vi ".....GAIT RECOGNITION only.vi"() -> ()   [LabVIEW 2018]
uses:
  <vilib>/University of Leeds/Kinesthesia Toolkit for Microsoft Kinect/_Polymorphic Configure/Event-Skeleton and Video.vi
  <vilib>/Utility/file.llb/Read Delimited Spreadsheet (DBL).vi
  <vilib>/University of Leeds/Kinesthesia Toolkit for Microsoft Kinect/_Polymorphic Read/Read-Skeleton and Video.vi
  <vilib>/University of Leeds/Kinesthesia Toolkit for Microsoft Kinect/_Polymorphic Close/Close-Skeleton and Video.vi
panel:
  out "3D Skeleton":refnum<vi>(3d-picture)
  out "2D Picture":picture
  out "recognized??":bool
  out "real time bone length":dbl[](array[numeric])
  out "19 means":dbl[][](array[numeric])
  in  "file path":path=path "D:/mean.csv"
  out "score":dbl
  # "Skeleton Recognition System"
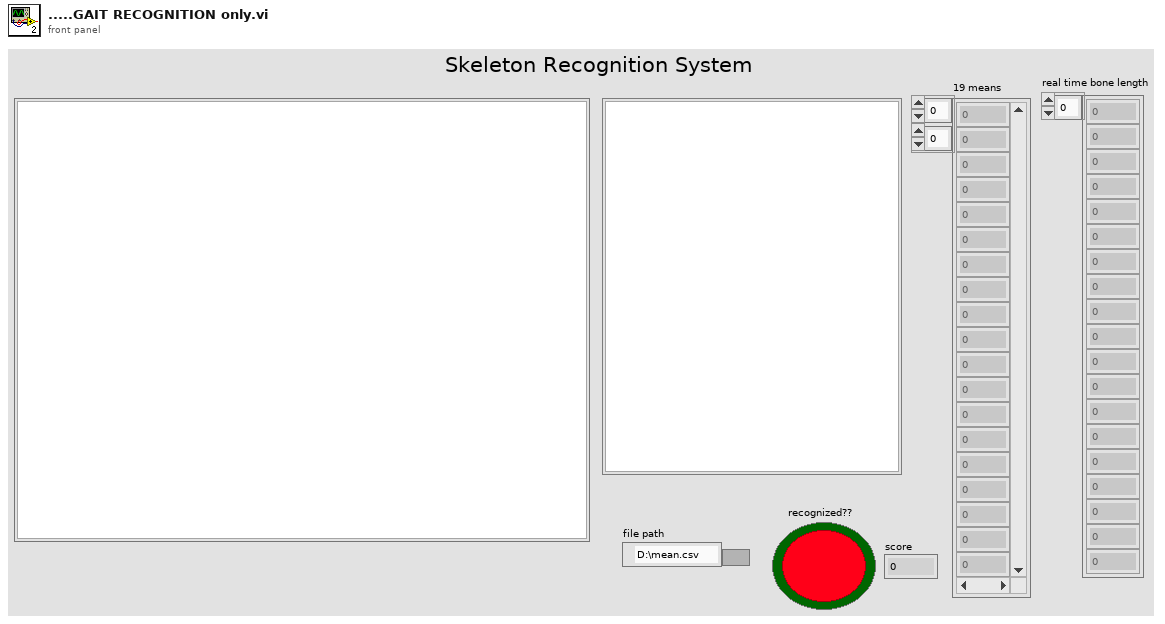
[diagram p1: front panel]
types:
  T1 = enum16{"hip centre", "spine", "shoulder centre", "head", "shoulder left", "elbow left", "wrist left", "hand left", "shoulder right", "elbow right", "wrist right", "hand right", "hip left", "knee left", "ankle left", "foot left", "hip right", "knee right", "ankle right", "foot right"}
  T2 = cluster{cluster{"reference out":refnum<k24>, "KinectSensors":refnum<k24>}, "get_Item":refnum<k24>}
  T3 = cluster{"reference out":refnum<k24>, "KinectSensors":refnum<k24>, "SkeletonStream":refnum<k24>, "ColorStream":refnum<k24>, refnum<k24>[], "get_Item":refnum<k24>}
  T4 = cluster{"Scene":refnum<vi>, "Joints":refnum<vi>[], "Bones":refnum<vi>[]}
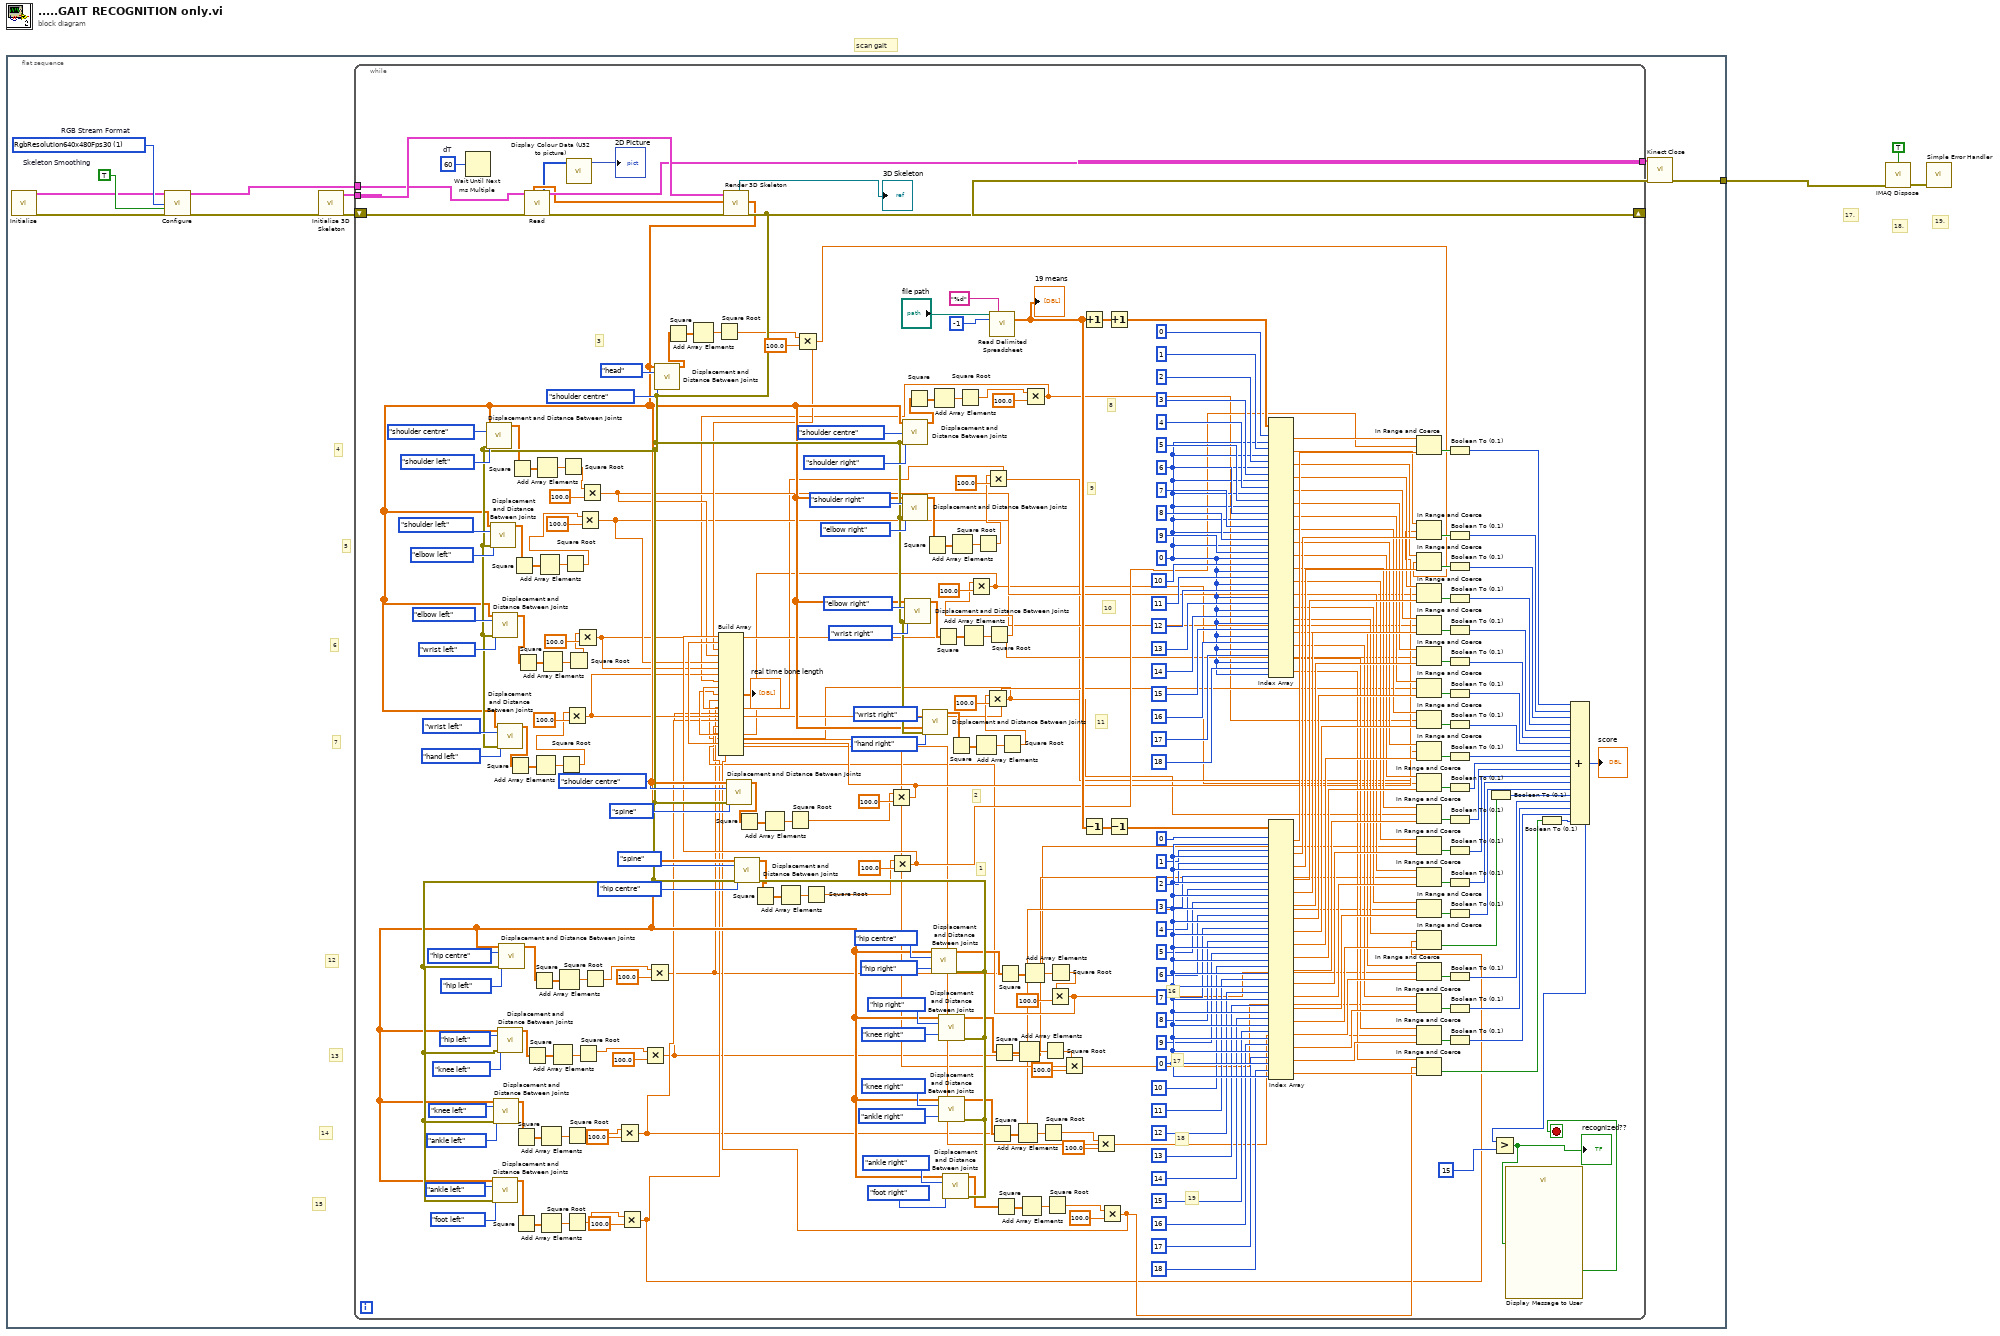
[diagram p0: block diagram]
diagram:
  # "19."
  # "17."
  # "18."
  # "scan gait"
  n1 = flat-sequence {
    tunnel: [w4] -> w1
    frame #0 {
      w10 = 1 items=["Undefined", "RgbResolution640x480Fps30", "RgbResolution1280x960Fps12", "YuvResolution640x480Fps15", "RawYuvResolution640x480Fps15"]  # RGB Stream Format
      w9 = TRUE  # Skeleton Smoothing
      # "15"
      # "14"
      # "13"
      # "12"
      # "7"
      # "6"
      # "5"
      # "4"
      n2 = call <vilib>:"Initialise.vi"() -> ("Kinect References out"=w5:T2, "error out"=w6:errorcluster)  [unwired: 14 in]
      n3 = call-poly <vilib>:"Configure.vi"("Kinect References in"=w5, "RGB Stream Format"=w10, "Skeleton Smoothing"=w9, "error in"=w6) -> ("Kinect References out"=w11:T3, "error out"=w12:errorcluster)  [unwired: 10 in]
      n4 = call <vilib>:"Initialise 3D Skeleton.vi"("error in (no error)"=w12) -> ("error out"=w13:errorcluster, "Scene & Skeleton Refs"=w14:T4)  [unwired: 9 in]
      n5 = while {
        tunnel: [w301] -> w7
        tunnel: w14 -> [w307]
        tunnel: w11 -> [w302]
        shift-right: [w260] -> w8
        shift-left: w13 -> [w304]
        stop <- w15 stop-if-true
        w136 = 0 ("disabled index (col)")
        w138 = 0 ("disabled index (col)")
        w305 = u32 60  # dT
        # "19"
        # "18"
        # "17"
        # "16"
        # "2"
        # "1"
        # "11"
        # "10"
        # "9"
        # "8"
        # "3"
        n6 = Wait Until Next ms Multiple(millisecond multiple=w305) -> ()  [unwired: 1 out]
        n7 = call-poly <vilib>:"Read.vi"("Kinect References in"=w302, "error in (no error)"=w304) -> ("Primary Skeleton Array"=w300:dbl[][], "Colour output array (U24, RGB)"=w299:u32[][], "Kinect References out"=w301:T3, "error out"=w303:errorcluster)  [unwired: 9 in, 1 out]
        n8 = call <vilib>:"Display Colour Data (U32 to picture).vi"("Colour output array (U24, RGB)"=w299) -> ("new picture"=→"2D Picture":picture)  [unwired: 10 in]
        n9 = call <vilib>:"Render 3D Skeleton.vi"("error in (no error)"=w303, "Array of Joint Positions"=w300, "Scene & Skeleton Refs In"=w307) -> ("error out"=w260:errorcluster, "Array of Joint Positions Out"=w259:dbl[][], "Scene Out"=→"3D Skeleton":refnum<vi>)  [unwired: 5 in, 1 out]
        n10 = call <vilib>:"Displacement and Distance Between Joints.vi"("Array of Joint Positions"=w259, "Joint 1"=T1."shoulder centre", "Joint 2"=T1."shoulder left", "error in (no error)"=w260) -> ("X Y Z Displacement Between Joints 1 and 2"=w250:dbl[])  [unwired: 10 in, 1 out]
        n11 = call <vilib>:"Displacement and Distance Between Joints.vi"("Array of Joint Positions"=w259, "Joint 1"=T1."shoulder left", "Joint 2"=T1."elbow left", "error in (no error)"=w260) -> ("X Y Z Displacement Between Joints 1 and 2"=w247:dbl[])  [unwired: 10 in, 1 out]
        n12 = call <vilib>:"Displacement and Distance Between Joints.vi"("Array of Joint Positions"=w259, "Joint 1"=T1."elbow left", "Joint 2"=T1."wrist left", "error in (no error)"=w260) -> ("X Y Z Displacement Between Joints 1 and 2"=w241:dbl[])  [unwired: 10 in, 1 out]
        n13 = call <vilib>:"Displacement and Distance Between Joints.vi"("Array of Joint Positions"=w259, "Joint 1"=T1."ankle left", "Joint 2"=T1."foot left", "error in (no error)"=w260) -> ("X Y Z Displacement Between Joints 1 and 2"=w214:dbl[])  [unwired: 10 in, 1 out]
        n14 = call <vilib>:"Displacement and Distance Between Joints.vi"("Array of Joint Positions"=w259, "Joint 1"=T1."knee left", "Joint 2"=T1."ankle left", "error in (no error)"=w260) -> ("X Y Z Displacement Between Joints 1 and 2"=w215:dbl[])  [unwired: 10 in, 1 out]
        n15 = call <vilib>:"Displacement and Distance Between Joints.vi"("Array of Joint Positions"=w259, "Joint 1"=T1."wrist left", "Joint 2"=T1."hand left", "error in (no error)"=w260) -> ("X Y Z Displacement Between Joints 1 and 2"=w231:dbl[])  [unwired: 10 in, 1 out]
        n16 = call <vilib>:"Displacement and Distance Between Joints.vi"("Array of Joint Positions"=w259, "Joint 1"=T1."hip left", "Joint 2"=T1."knee left", "error in (no error)"=w260) -> ("X Y Z Displacement Between Joints 1 and 2"=w216:dbl[])  [unwired: 10 in, 1 out]
        n17 = call <vilib>:"Displacement and Distance Between Joints.vi"("Array of Joint Positions"=w259, "Joint 1"=T1."hip centre", "Joint 2"=T1."hip left", "error in (no error)"=w260) -> ("X Y Z Displacement Between Joints 1 and 2"=w223:dbl[])  [unwired: 10 in, 1 out]
        n18 = Square(x=w231) -> (x^2=w235:dbl[])
        n19 = Square(x=w250) -> (x^2=w252:dbl[])
        n20 = Square(x=w247) -> (x^2=w249:dbl[])
        n21 = Square(x=w215) -> (x^2=w220:dbl[])
        n22 = Square(x=w214) -> (x^2=w218:dbl[])
        n23 = Square(x=w241) -> (x^2=w243:dbl[])
        n24 = Square(x=w216) -> (x^2=w222:dbl[])
        n25 = Square(x=w223) -> (x^2=w225:dbl[])
        n26 = Add Array Elements(numeric array=w235) -> (sum=w234:dbl)
        n27 = Add Array Elements(numeric array=w252) -> (sum=w251:dbl)
        n28 = Add Array Elements(numeric array=w249) -> (sum=w248:dbl)
        n29 = Add Array Elements(numeric array=w220) -> (sum=w219:dbl)
        n30 = Add Array Elements(numeric array=w218) -> (sum=w217:dbl)
        n31 = Add Array Elements(numeric array=w243) -> (sum=w242:dbl)
        n32 = Add Array Elements(numeric array=w222) -> (sum=w221:dbl)
        n33 = Add Array Elements(numeric array=w225) -> (sum=w224:dbl)
        n34 = Square Root(x=w234) -> (sqrt(x)=w190:dbl)
        n35 = Square Root(x=w251) -> (sqrt(x)=w198:dbl)
        n36 = Square Root(x=w248) -> (sqrt(x)=w194:dbl)
        n37 = Multiply(x=w190, y=100.0) -> (x*y=w29:dbl)
        n38 = Square Root(x=w219) -> (sqrt(x)=w172:dbl)
        n39 = Square Root(x=w217) -> (sqrt(x)=w170:dbl)
        n40 = Square Root(x=w242) -> (sqrt(x)=w192:dbl)
        n41 = Multiply(x=w192, y=100.0) -> (x*y=w30:dbl)
        n42 = Square Root(x=w221) -> (sqrt(x)=w174:dbl)
        n43 = Multiply(x=w194, y=100.0) -> (x*y=w31:dbl)
        n44 = Multiply(x=w198, y=100.0) -> (x*y=w32:dbl)
        n45 = Square Root(x=w224) -> (sqrt(x)=w176:dbl)
        n46 = Multiply(x=w172, y=100.0) -> (x*y=w20:dbl)
        n47 = Multiply(x=w170, y=100.0) -> (x*y=w21:dbl)
        n48 = Multiply(x=w174, y=100.0) -> (x*y=w19:dbl)
        n49 = Multiply(x=w176, y=100.0) -> (x*y=w18:dbl)
        n50 = call <vilib>:"Displacement and Distance Between Joints.vi"("Array of Joint Positions"=w259, "Joint 1"=T1."head", "Joint 2"=T1."shoulder centre", "error in (no error)"=w260) -> ("X Y Z Displacement Between Joints 1 and 2"=w256:dbl[])  [unwired: 10 in, 1 out]
        n51 = Square(x=w256) -> (x^2=w258:dbl[])
        n52 = Add Array Elements(numeric array=w258) -> (sum=w257:dbl)
        n53 = Square Root(x=w257) -> (sqrt(x)=w196:dbl)
        n54 = call <vilib>:"Displacement and Distance Between Joints.vi"("Array of Joint Positions"=w259, "Joint 1"=T1."shoulder centre", "Joint 2"=T1."spine", "error in (no error)"=w260) -> ("X Y Z Displacement Between Joints 1 and 2"=w229:dbl[])  [unwired: 10 in, 1 out]
        n55 = call <vilib>:"Displacement and Distance Between Joints.vi"("Array of Joint Positions"=w259, "Joint 1"=T1."spine", "Joint 2"=T1."hip centre", "error in (no error)"=w260) -> ("X Y Z Displacement Between Joints 1 and 2"=w226:dbl[])  [unwired: 10 in, 1 out]
        n56 = Square(x=w229) -> (x^2=w237:dbl[])
        n57 = Square(x=w226) -> (x^2=w228:dbl[])
        n58 = Add Array Elements(numeric array=w237) -> (sum=w236:dbl)
        n59 = Add Array Elements(numeric array=w228) -> (sum=w227:dbl)
        n60 = Square Root(x=w236) -> (sqrt(x)=w188:dbl)
        n61 = Multiply(x=w196, y=100.0) -> (x*y=w33:dbl)
        n62 = Square Root(x=w227) -> (sqrt(x)=w178:dbl)
        n63 = Multiply(x=w188, y=100.0) -> (x*y=w34:dbl)
        n64 = Multiply(x=w178, y=100.0) -> (x*y=w35:dbl)
        n65 = call <vilib>:"Displacement and Distance Between Joints.vi"("Array of Joint Positions"=w259, "Joint 1"=T1."shoulder centre", "Joint 2"=T1."shoulder right", "error in (no error)"=w260) -> ("X Y Z Displacement Between Joints 1 and 2"=w253:dbl[])  [unwired: 10 in, 1 out]
        n66 = call <vilib>:"Displacement and Distance Between Joints.vi"("Array of Joint Positions"=w259, "Joint 1"=T1."shoulder right", "Joint 2"=T1."elbow right", "error in (no error)"=w260) -> ("X Y Z Displacement Between Joints 1 and 2"=w244:dbl[])  [unwired: 10 in, 1 out]
        n67 = call <vilib>:"Displacement and Distance Between Joints.vi"("Array of Joint Positions"=w259, "Joint 1"=T1."elbow right", "Joint 2"=T1."wrist right", "error in (no error)"=w260) -> ("X Y Z Displacement Between Joints 1 and 2"=w238:dbl[])  [unwired: 10 in, 1 out]
        n68 = Square(x=w253) -> (x^2=w255:dbl[])
        n69 = call <vilib>:"Displacement and Distance Between Joints.vi"("Array of Joint Positions"=w259, "Joint 1"=T1."wrist right", "Joint 2"=T1."hand right", "error in (no error)"=w260) -> ("X Y Z Displacement Between Joints 1 and 2"=w230:dbl[])  [unwired: 10 in, 1 out]
        n70 = Square(x=w244) -> (x^2=w246:dbl[])
        n71 = Add Array Elements(numeric array=w255) -> (sum=w254:dbl)
        n72 = call <vilib>:"Displacement and Distance Between Joints.vi"("Array of Joint Positions"=w259, "Joint 1"=T1."hip centre", "Joint 2"=T1."hip right", "error in (no error)"=w260) -> ("X Y Z Displacement Between Joints 1 and 2"=w211:dbl[])  [unwired: 10 in, 1 out]
        n73 = Square(x=w238) -> (x^2=w240:dbl[])
        n74 = call <vilib>:"Displacement and Distance Between Joints.vi"("Array of Joint Positions"=w259, "Joint 1"=T1."hip right", "Joint 2"=T1."knee right", "error in (no error)"=w260) -> ("X Y Z Displacement Between Joints 1 and 2"=w204:dbl[])  [unwired: 10 in, 1 out]
        n75 = call <vilib>:"Displacement and Distance Between Joints.vi"("Array of Joint Positions"=w259, "Joint 1"=T1."knee right", "Joint 2"=T1."ankle right", "error in (no error)"=w260) -> ("X Y Z Displacement Between Joints 1 and 2"=w203:dbl[])  [unwired: 10 in, 1 out]
        n76 = call <vilib>:"Displacement and Distance Between Joints.vi"("Array of Joint Positions"=w259, "Joint 1"=T1."ankle right", "Joint 2"=T1."foot right", "error in (no error)"=w260) -> ("X Y Z Displacement Between Joints 1 and 2"=w202:dbl[])  [unwired: 10 in, 1 out]
        n77 = Square(x=w230) -> (x^2=w233:dbl[])
        n78 = Add Array Elements(numeric array=w246) -> (sum=w245:dbl)
        n79 = Square Root(x=w254) -> (sqrt(x)=w186:dbl)
        n80 = Add Array Elements(numeric array=w240) -> (sum=w239:dbl)
        n81 = Add Array Elements(numeric array=w233) -> (sum=w232:dbl)
        n82 = Square Root(x=w245) -> (sqrt(x)=w184:dbl)
        n83 = Multiply(x=w184, y=100.0) -> (x*y=w27:dbl)
        n84 = Square Root(x=w239) -> (sqrt(x)=w182:dbl)
        n85 = Multiply(x=w182, y=100.0) -> (x*y=w26:dbl)
        n86 = call-poly <vilib>:"Read Delimited Spreadsheet.vi"("file path (dialog if empty)"="file path", "format (%.3f)"="%d", "number of rows (all:-1)"=-1) -> ("all rows"=w114:dbl[][])  [unwired: 7 in, 5 out]
        "19 means" <- w114
        n87 = Square(x=w203) -> (x^2=w208:dbl[])
        n88 = Square(x=w204) -> (x^2=w210:dbl[])
        n89 = Square(x=w202) -> (x^2=w205:dbl[])
        n90 = Square(x=w211) -> (x^2=w213:dbl[])
        n91 = Square Root(x=w232) -> (sqrt(x)=w180:dbl)
        n92 = Multiply(x=w180, y=100.0) -> (x*y=w17:dbl)
        n93 = Add Array Elements(numeric array=w208) -> (sum=w207:dbl)
        n94 = Add Array Elements(numeric array=w210) -> (sum=w209:dbl)
        n95 = Add Array Elements(numeric array=w205) -> (sum=w206:dbl)
        n96 = Add Array Elements(numeric array=w213) -> (sum=w212:dbl)
        n97 = Multiply(x=w186, y=100.0) -> (x*y=w28:dbl)
        n98 = Square Root(x=w207) -> (sqrt(x)=w166:dbl)
        n99 = Square Root(x=w209) -> (sqrt(x)=w164:dbl)
        n100 = Square Root(x=w206) -> (sqrt(x)=w168:dbl)
        n101 = Square Root(x=w212) -> (sqrt(x)=w162:dbl)
        n102 = Multiply(x=w162, y=100.0) -> (x*y=w22:dbl)
        n103 = Multiply(x=w164, y=100.0) -> (x*y=w23:dbl)
        n104 = Increment(x=w114) -> (x+1=w113:dbl[][])
        n105 = Decrement(x=w114) -> (x-1=w115:dbl[][])
        n106 = Multiply(x=w166, y=100.0) -> (x*y=w24:dbl)
        n107 = Multiply(x=w168, y=100.0) -> (x*y=w25:dbl)
        n108 = Build Array(w35, w34, w33, w32, w31, w30, w29, w28, w27, w26, w17, w18, w19, w20, w21, w22, w23, w24, w25) -> (→"real time bone length":dbl[])
        n109 = Increment(x=w113) -> (x+1=w137:dbl[][])
        n110 = Decrement(x=w115) -> (x-1=w116:dbl[][])
        n111 = Index Array(array=w137, index (row) #1=0 ("disabled index (row)"), index (col) #1=w138, index (row) #2=1 ("disabled index (row)"), index (col) #2=w138, index (row) #3=2 ("disabled index (row)"), index (col) #3=w138, index (row) #4=3 ("disabled index (row)"), index (col) #4=w138, index (row) #5=4 ("disabled index (row)"), index (col) #5=w138, index (row) #6=5 ("disabled index (row)"), index (col) #6=w138, index (row) #7=6 ("disabled index (row)"), index (col) #7=w138, index (row) #8=7 ("disabled index (row)"), index (col) #8=w138, index (row) #9=8 ("disabled index (row)"), index (col) #9=w138, index (row) #10=9 ("disabled index (row)"), index (col) #10=w138, index (row) #11=10 ("disabled index (row)"), index (col) #11=w138, index (row) #12=11 ("disabled index (row)"), index (col) #12=w138, index (row) #13=12 ("disabled index (row)"), index (col) #13=w138, index (row) #14=13 ("disabled index (row)"), index (col) #14=w138, index (row) #15=14 ("disabled index (row)"), index (col) #15=w138, index (row) #16=15 ("disabled index (row)"), index (col) #16=w138, index (row) #17=16 ("disabled index (row)"), index (col) #17=w138, index (row) #18=17 ("disabled index (row)"), index (col) #18=w138, index (row) #19=18 ("disabled index (row)"), index (col) #19=w138) -> (element #1=w76:dbl, element #2=w56:dbl, element #3=w55:dbl, element #4=w54:dbl, element #5=w53:dbl, element #6=w52:dbl, element #7=w51:dbl, element #8=w50:dbl, element #9=w49:dbl, element #10=w48:dbl, element #11=w39:dbl, element #12=w40:dbl, element #13=w41:dbl, element #14=w42:dbl, element #15=w43:dbl, element #16=w44:dbl, element #17=w45:dbl, element #18=w46:dbl, element #19=w47:dbl)
        n112 = Index Array(array=w116, index (row) #1=0 ("disabled index (row)"), index (col) #1=w136, index (row) #2=1 ("disabled index (row)"), index (col) #2=w136, index (row) #3=2 ("disabled index (row)"), index (col) #3=w136, index (row) #4=3 ("disabled index (row)"), index (col) #4=w136, index (row) #5=4 ("disabled index (row)"), index (col) #5=w136, index (row) #6=5 ("disabled index (row)"), index (col) #6=w136, index (row) #7=6 ("disabled index (row)"), index (col) #7=w136, index (row) #8=7 ("disabled index (row)"), index (col) #8=w136, index (row) #9=8 ("disabled index (row)"), index (col) #9=w136, index (row) #10=9 ("disabled index (row)"), index (col) #10=w136, index (row) #11=10 ("disabled index (row)"), index (col) #11=w136, index (row) #12=11 ("disabled index (row)"), index (col) #12=w136, index (row) #13=12 ("disabled index (row)"), index (col) #13=w136, index (row) #14=13 ("disabled index (row)"), index (col) #14=w136, index (row) #15=14 ("disabled index (row)"), index (col) #15=w136, index (row) #16=15 ("disabled index (row)"), index (col) #16=w136, index (row) #17=16 ("disabled index (row)"), index (col) #17=w136, index (row) #18=17 ("disabled index (row)"), index (col) #18=w136, index (row) #19=18 ("disabled index (row)"), index (col) #19=w136) -> (element #1=w75:dbl, element #2=w74:dbl, element #3=w73:dbl, element #4=w72:dbl, element #5=w71:dbl, element #6=w70:dbl, element #7=w69:dbl, element #8=w68:dbl, element #9=w67:dbl, element #10=w66:dbl, element #11=w65:dbl, element #12=w64:dbl, element #13=w63:dbl, element #14=w62:dbl, element #15=w61:dbl, element #16=w60:dbl, element #17=w59:dbl, element #18=w58:dbl, element #19=w57:dbl)
        n113 = In Range and Coerce(upper limit=w76, x=w35, lower limit=w75) -> (In Range?=w112:bool)  [unwired: 1 out]
        n114 = In Range and Coerce(upper limit=w56, x=w34, lower limit=w74) -> (In Range?=w111:bool)  [unwired: 1 out]
        n115 = In Range and Coerce(upper limit=w55, x=w33, lower limit=w73) -> (In Range?=w110:bool)  [unwired: 1 out]
        n116 = In Range and Coerce(upper limit=w54, x=w32, lower limit=w72) -> (In Range?=w109:bool)  [unwired: 1 out]
        n117 = In Range and Coerce(upper limit=w53, x=w31, lower limit=w71) -> (In Range?=w108:bool)  [unwired: 1 out]
        n118 = In Range and Coerce(upper limit=w52, x=w30, lower limit=w70) -> (In Range?=w107:bool)  [unwired: 1 out]
        n119 = In Range and Coerce(upper limit=w51, x=w29, lower limit=w69) -> (In Range?=w106:bool)  [unwired: 1 out]
        n120 = In Range and Coerce(upper limit=w50, x=w28, lower limit=w68) -> (In Range?=w105:bool)  [unwired: 1 out]
        n121 = In Range and Coerce(upper limit=w49, x=w27, lower limit=w67) -> (In Range?=w104:bool)  [unwired: 1 out]
        n122 = In Range and Coerce(upper limit=w48, x=w26, lower limit=w66) -> (In Range?=w103:bool)  [unwired: 1 out]
        n123 = In Range and Coerce(upper limit=w39, x=w17, lower limit=w65) -> (In Range?=w102:bool)  [unwired: 1 out]
        n124 = In Range and Coerce(upper limit=w40, x=w18, lower limit=w64) -> (In Range?=w101:bool)  [unwired: 1 out]
        n125 = In Range and Coerce(upper limit=w41, x=w19, lower limit=w63) -> (In Range?=w100:bool)  [unwired: 1 out]
        n126 = In Range and Coerce(upper limit=w42, x=w20, lower limit=w62) -> (In Range?=w99:bool)  [unwired: 1 out]
        n127 = In Range and Coerce(upper limit=w43, x=w21, lower limit=w61) -> (In Range?=w37:bool)  [unwired: 1 out]
        n128 = In Range and Coerce(upper limit=w44, x=w22, lower limit=w60) -> (In Range?=w98:bool)  [unwired: 1 out]
        n129 = In Range and Coerce(upper limit=w45, x=w23, lower limit=w59) -> (In Range?=w97:bool)  [unwired: 1 out]
        n130 = In Range and Coerce(upper limit=w46, x=w24, lower limit=w58) -> (In Range?=w96:bool)  [unwired: 1 out]
        n131 = In Range and Coerce(upper limit=w47, x=w25, lower limit=w57) -> (In Range?=w38:bool)  [unwired: 1 out]
        n132 = Boolean To (0,1)(Boolean=w112) -> (0, 1=w95:i16)
        n133 = Boolean To (0,1)(Boolean=w111) -> (0, 1=w94:i16)
        n134 = Boolean To (0,1)(Boolean=w110) -> (0, 1=w93:i16)
        n135 = Boolean To (0,1)(Boolean=w109) -> (0, 1=w92:i16)
        n136 = Boolean To (0,1)(Boolean=w108) -> (0, 1=w91:i16)
        n137 = Boolean To (0,1)(Boolean=w107) -> (0, 1=w90:i16)
        n138 = Boolean To (0,1)(Boolean=w106) -> (0, 1=w89:i16)
        n139 = Boolean To (0,1)(Boolean=w105) -> (0, 1=w88:i16)
        n140 = Boolean To (0,1)(Boolean=w104) -> (0, 1=w87:i16)
        n141 = Boolean To (0,1)(Boolean=w103) -> (0, 1=w86:i16)
        n142 = Boolean To (0,1)(Boolean=w102) -> (0, 1=w85:i16)
        n143 = Boolean To (0,1)(Boolean=w101) -> (0, 1=w84:i16)
        n144 = Boolean To (0,1)(Boolean=w100) -> (0, 1=w83:i16)
        n145 = Boolean To (0,1)(Boolean=w99) -> (0, 1=w82:i16)
        n146 = Boolean To (0,1)(Boolean=w98) -> (0, 1=w80:i16)
        n147 = Boolean To (0,1)(Boolean=w97) -> (0, 1=w79:i16)
        n148 = Boolean To (0,1)(Boolean=w96) -> (0, 1=w78:i16)
        n149 = Boolean To (0,1)(Boolean=w37) -> (0, 1=w81:i16)
        n150 = Boolean To (0,1)(Boolean=w38) -> (0, 1=w77:i16)
        n151 = Compound Arithmetic op=ADD(w95, w94, w93, w92, w91, w90, w89, w88, w87, w86, w85, w84, w83, w82, w81, w80, w79, w78, w77) -> (w36:i16)
        "score" <- w36
        n152 = Greater?(x=w36, y=i16 15) -> (0:w16:bool)
        "recognized??" <- w16
        n153 = call "Display Message to User"("Enable"=w16) -> ("OK"=w15:bool)  [unwired: 9 in, 1 out]
      }
      n154 = call-poly <vilib>:"Kinect Close.vi"("Kinect References in"=w7, "error in"=w8) -> ("error out"=w4:errorcluster)  [unwired: 13 in]
    }
  }
  n155 = call "IMAQ Dispose"("All Images? (No)"=TRUE, "error in (no error)"=w1) -> ("error out"=w3:errorcluster)  [unwired: 1 in, 3 out]
  n156 = call <vilib>:"Simple Error Handler.vi"("error in (no error)"=w3) -> ()  [unwired: 1 in, 8 out]
